vi "UpdaeCoorOverlay.vi"(5 "ImageCtl":refnum<vi>, 7 "CoordinatePoints":refnum<vi>, 11 "Image":T1) -> (3 "Image Out":T1)   [LabVIEW 2019]
uses:
  <vilib>/vision/Image Controls.llb/IMAQ Image.ctl
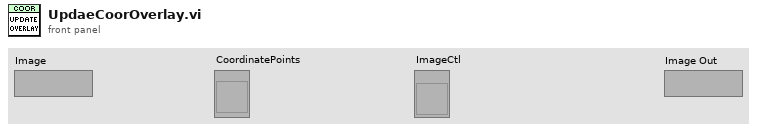
[diagram p1: front panel]
types:
  T1 = typedef "IMAQ Image.ctl" = refnum<image>
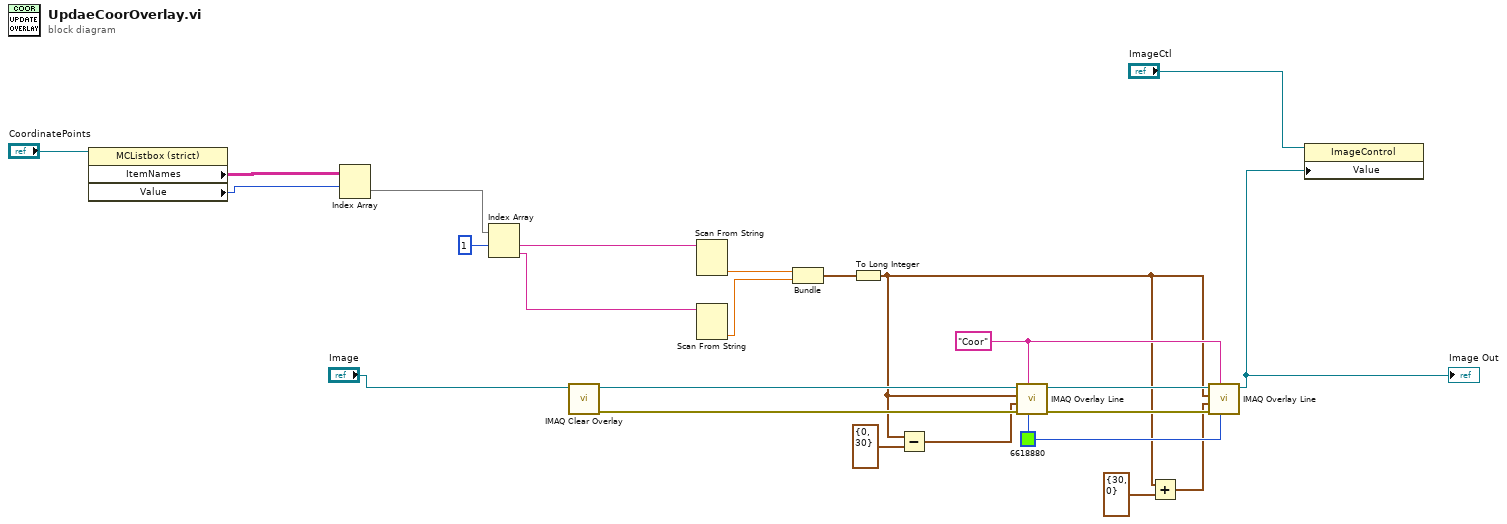
[diagram p0: block diagram]
diagram:
  w3 = "Coor" ("Group")
  w14 = u32 6618880 ("Color")
  n1 = property class="MCListbox (strict)"(reference="CoordinatePoints") -> ("ItemNames"=w8:string[][], "Value"=w4:i32)  [unwired: 1 in, 2 out]
  n2 = Index Array(array=w8, index (row)=w4) -> (element=w5:string[])  [unwired: 1 in]
  n3 = Index Array(array=w5, index #1=1 ("index")) -> (element #1=w22:string, element #2=w21:string)  [unwired: 1 in]
  n4 = call "IMAQ Clear Overlay"("Image"="Image") -> ("error out"=w16:errorcluster, "Image Out"=w17:T1)  [unwired: 9 in]
  n5 = Scan From String(input string=w22) -> (output 1=w20:dbl)  [unwired: 4 in, 3 out]
  n6 = Scan From String(input string=w21) -> (output 1=w19:dbl)  [unwired: 4 in, 3 out]
  n7 = Bundle(w20, w19) -> (w18:cluster{dbl, dbl})  [unwired: 1 in]
  n8 = To Long Integer(number=w18) -> (32bit integer=w2:cluster{i32, i32})
  n9 = Subtract(x=w2, y=cluster{i32, i32} {0, 30}) -> (x-y=w12:cluster{i32, i32})
  n10 = call "IMAQ Overlay Line"("Color"=w14, "Group"=w3, "error in (no error)"=w16, "End Point"=w12, "Start Point"=w2, "Image"=w17) -> ("error out"=w13:errorcluster, "Image Out"=w15:T1)  [unwired: 4 in]
  n11 = Add(x=w2, y=cluster{i32, i32} {30, 0}) -> (x+y=w10:cluster{i32, i32})
  n12 = call "IMAQ Overlay Line"("Color"=w14, "Group"=w3, "error in (no error)"=w13, "End Point"=w10, "Start Point"=w2, "Image"=w15) -> ("Image Out"=w6:T1)  [unwired: 4 in, 1 out]
  "Image Out" <- w6
  n13 = property class="ImageControl"(reference="ImageCtl", "Value"=w6) -> ()  [unwired: 1 in, 2 out]
